vi "EV05故障解析.vi"() -> ()   [LabVIEW 2013]
panel:
  in  "选择故障类型":u32(ring) items=["电池故障", "硬件故障", "电池系统故障1", "电池系统故障2"]
  in  "输入故障码":string caption="输入故障码  (16位的十六进制数值)"
  in  "故码障解析123":bool
  out "电池故障":string[][](array[string])
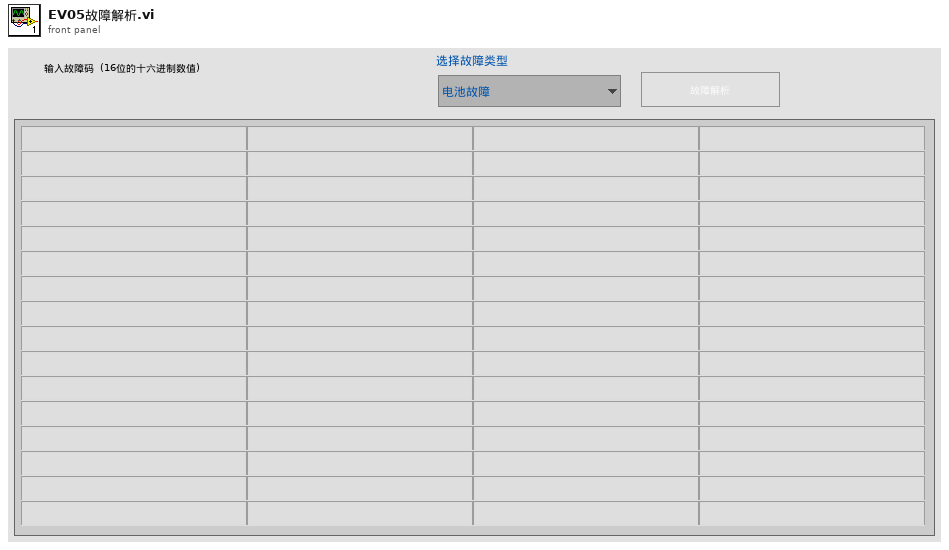
[diagram p1: front panel]
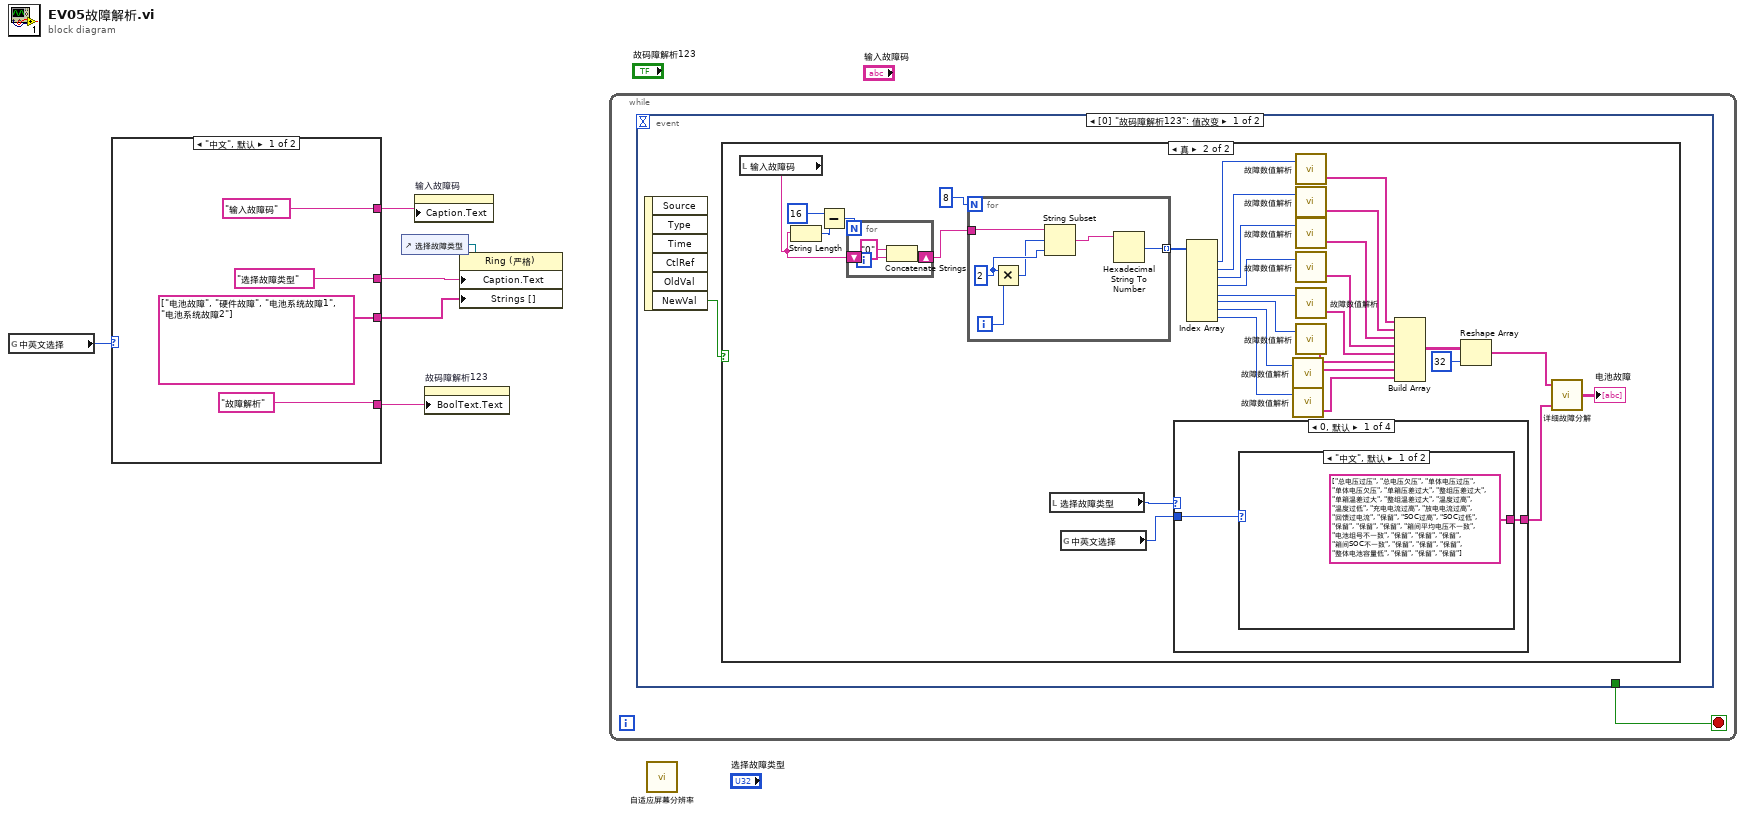
[diagram p0: block diagram]
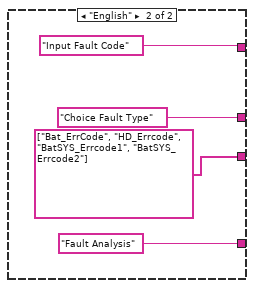
[diagram p2: hidden frame]
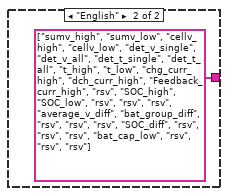
[diagram p4: hidden frame]
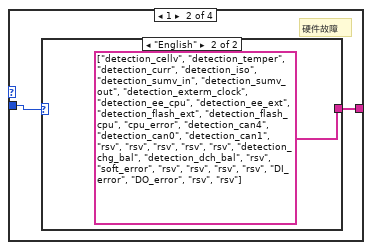
[diagram p5: hidden frame]
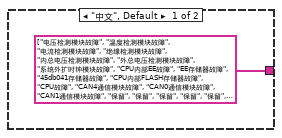
[diagram p6: hidden frame]
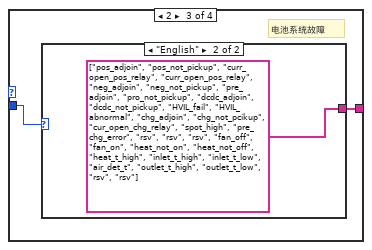
[diagram p7: hidden frame]
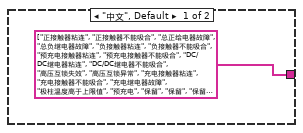
[diagram p8: hidden frame]
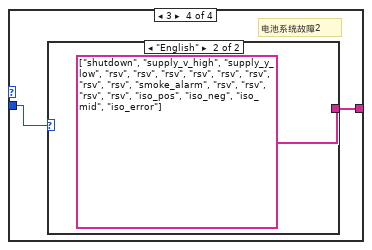
[diagram p9: hidden frame]
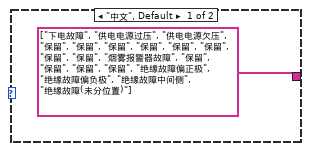
[diagram p10: hidden frame]
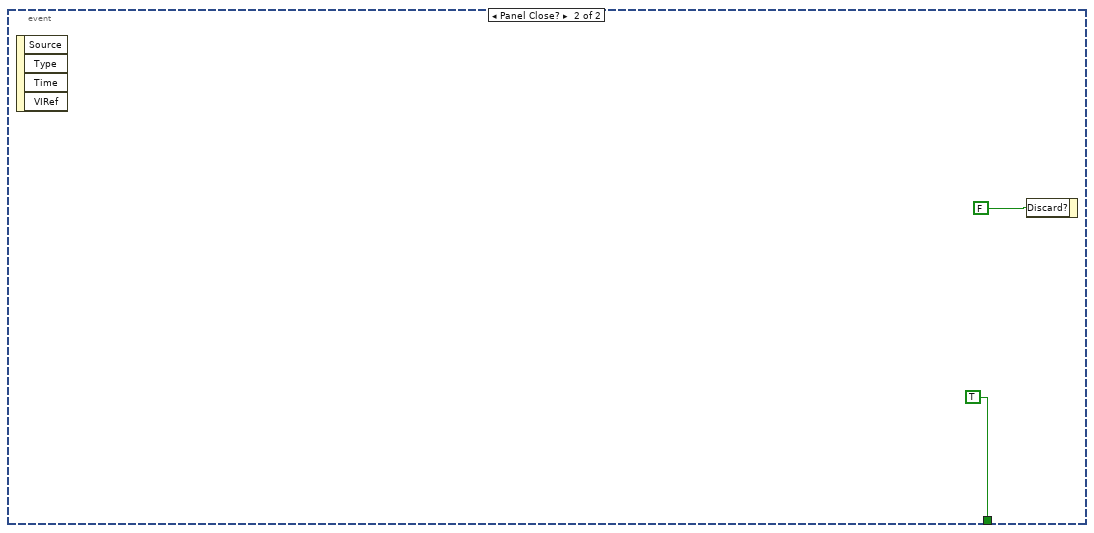
[diagram p11: hidden frame]
diagram:
  n1 = global read "中英文全局.vi" "中英文选择"() -> (w1:enum32{"中文", "English"})
  n2 = case shown="\"中文\", 默认" w1 {
    tunnel: ["输入故障码" "Input Fault Code"] -> w6
    tunnel: ["选择故障类型" "Choice Fault Type"] -> w4
    tunnel: [string[] ["电池故障", "硬件故障", "电池系统故障1", "电池系统故障2"] ("字符串[]") string[] ["Bat_ErrCode", "HD_Errcode", "BatSYS_Errcode1", "BatSYS_Errcode2"] ("字符串[]")] -> w3
    tunnel: ["故障解析" "Fault Analysis"] -> w2
    frame "中文", Default {
    }
    frame "English" {
    }
  }
  n3 = control-ref of="选择故障类型"() -> (w5:refnum<vi>)
  n4 = property on="输入故障码" class="Str"("Caption.Text"=w6) -> ()  [unwired: 2 in, 2 out]
  n5 = property on="故码障解析123" class="Bool (严格)"("BoolText.Text"=w2) -> ()  [unwired: 2 in, 2 out]
  n6 = property class="Ring (严格)"(reference=w5, "Caption.Text"=w4, "Strings []"=w3) -> ()  [unwired: 1 in, 2 out]
  n7 = while {
    stop <- w15 stop-if-true
    n8 = event shown="[0] \"故码障解析123\": 值改变" {
      selector: _ -> [_ _]
      dyn-events: _ -> [_ _]
      timeout: _ -> [_ _]
      tunnel: [_ TRUE] -> w15
      event "故码障解析123": Value Change {
        n9 = event-data() -> ("NewVal"=w16:bool)  [unwired: 1 in, 5 out]
        n10 = case shown="真" w16 {
          frame False {
          }
          frame True {
            n11 = local read "输入故障码"() -> (w19:string)
            n12 = String Length(string=w19) -> (length=w21:i32)
            n13 = Subtract(x=16, y=w21) -> (x-y=w23:i32)
            n14 = for {
              N: w23 -> [_]
              shift-right: [w47] -> w20
              shift-left: w19 -> [w49]
              n15 = Concatenate Strings("0" ("字符串"), w49) -> (w47:string)
            }
            n16 = for {
              N: 8 -> [_]
              tunnel: w20 -> [w55]
              tunnel: [w54] -> w34 mode=indexing
              i -> [w50]
              w52 = 2 ("x")
              n17 = Multiply(x=w52, y=w50) -> (x*y=w51:i32)
              n18 = String Subset(string=w55, offset (0)=w51, length (rest)=w52) -> (substring=w53:string)
              n19 = Hexadecimal String To Number(string=w53) -> (number=w54:u32)  [unwired: 2 in, 1 out]
            }
            n20 = local read "选择故障类型"() -> (w18:u32)
            n21 = global read "中英文全局.vi" "中英文选择"() -> (w17:enum32{"中文", "English"})
            n22 = case shown="0, 默认" w18 {
              tunnel: [w57 w61 w65 w69] -> w46
              tunnel: w17 -> [w56 w60 w64 w68]
              frame 0, Default {
                n23 = case shown="\"中文\", 默认" w56 {
                  tunnel: [string[] ["总电压过压", "总电压欠压", "单体电压过压", "单体电压欠压", "单箱压差过大", "整组压差过大", "单箱温差过大", "整组温差过大", "温度过高", "温度过低", "充电电流过高", "放电电流过高", "回馈过电流", "保留", "SOC过高", "SOC过低", "保留", "保留", "保留", "箱间平均电压不一致", "电池组号不一致", "保留", "保留", "保留", "箱间SOC不一致", "保留", "保留", "保留", "整体电池容量低", "保留", "保留", "保留"] ("名称") string[] ["sumv_high", "sumv_low", "cellv_high", "cellv_low", "det_v_single", "det_v_all", "det_t_single", "det_t_all", "t_high", "t_low", "chg_curr_high", "dch_curr_high", "Feedback_curr_high", "rsv", "SOC_high", "SOC_low", "rsv", "rsv", "rsv", "average_v_diff", "bat_group_diff", "rsv", "rsv", "rsv", "SOC_diff", "rsv", "rsv", "rsv", "bat_cap_low", "rsv", "rsv", "rsv"] ("名称")] -> w57
                  frame "中文", Default {
                  }
                  frame "English" {
                  }
                }
              }
              frame 1 {
                # "硬件故障"
                n24 = case shown="\"English\"" w60 {
                  tunnel: [string[] ["电压检测模块故障", "温度检测模块故障", "电流检测模块故障", "绝缘检测模块故障", "内总电压检测模块故障", "外总电压检测模块故障", "系统外扩时钟模块故障", "CPU内部EE故障", "EE存储器故障", "45db041存储器故障", "CPU内部FLASH存储器故障", "CPU故障", "CAN4通信模块故障", "CAN0通信模块故障", "CAN1通信模块故障", "保留", "保留", "保留", "保留", "保留", "充电均衡模块故障", "放电均衡模块故障", "保留", "软件故障", "保留", "保留", "保留", "保留", "DI模块故障", "DO模块故障", "保留", "保留"] ("名称") string[] ["detection_cellv", "detection_temper", "detection_curr", "detection_iso", "detection_sumv_in", "detection_sumv_out", "detection_exterm_clock", "detection_ee_cpu", "detection_ee_ext", "detection_flash_ext", "detection_flash_cpu", "cpu_error", "detection_can4", "detection_can0", "detection_can1", "rsv", "rsv", "rsv", "rsv", "rsv", "detection_chg_bal", "detection_dch_bal", "rsv", "soft_error", "rsv", "rsv", "rsv", "rsv", "DI_error", "DO_error", "rsv", "rsv"] ("名称")] -> w61
                  frame "中文", Default {
                  }
                  frame "English" {
                  }
                }
              }
              frame 2 {
                # "电池系统故障"
                n25 = case shown="\"English\"" w64 {
                  tunnel: [string[] ["正接触器粘连", "正接触器不能吸合", "总正给电器故障", "总负继电器故障", "负接触器粘连", "负接触器不能吸合", "预充电接触器粘连", "预充电接触器不能吸合", "DC/DC继电器粘连", "DC/DC继电器不能吸合", "高压互锁失效", "高压互锁异常", "充电接触器粘连", "充电接触器不能吸合", "充电继电器故障", "极柱温度高于上限值", "预充电", "保留", "保留", "保留", "风机堵路", "风机开路", "加热不能开启", "加热不能关闭", "加热器温度高于上限值", "进风口温度过高", "进风口温度过低", "进风口,出风口温差故障", "出风口温度过高", "出风口温度过低", "保留", "保留"] ("名称") string[] ["pos_adjoin", "pos_not_pickup", "curr_open_pos_relay", "curr_open_pos_relay", "neg_adjoin", "neg_not_pickup", "pre_adjoin", "pro_not_pickup", "dcdc_adjoin", "dcdc_not_pickup", "HVIL_fail", "HVIL_abnormal", "chg_adjoin", "chg_not_pcikup", "cur_open_chg_relay", "spot_high", "pre_chg_error", "rsv", "rsv", "rsv", "fan_off", "fan_on", "heat_not_on", "heat_not_off", "heat_t_high", "inlet_t_high", "inlet_t_low", "air_det_t", "outlet_t_high", "outlet_t_low", "rsv", "rsv"] ("名称")] -> w65
                  frame "中文", Default {
                  }
                  frame "English" {
                  }
                }
              }
              frame 3 {
                # "电池系统故障2"
                n26 = case shown="\"English\"" w68 {
                  tunnel: [string[] ["下电故障", "供电电源过压", "供电电源欠压", "保留", "保留", "保留", "保留", "保留", "保留", "保留", "保留", "烟雾报警器故障", "保留", "保留", "保留", "保留", "绝缘故障偏正极", "绝缘故障偏负极", "绝缘故障中间侧", "绝缘故障(未分位置)"] ("名称") string[] ["shutdown", "supply_v_high", "supply_y_low", "rsv", "rsv", "rsv", "rsv", "rsv", "rsv", "rsv", "rsv", "smoke_alarm", "rsv", "rsv", "rsv", "rsv", "iso_pos", "iso_neg", "iso_mid", "iso_error"] ("名称")] -> w69
                  frame "中文", Default {
                  }
                  frame "English" {
                  }
                }
              }
            }
            n27 = Index Array(array=w34) -> (element #1=w33:u32, element #2=w32:u32, element #3=w31:u32, element #4=w30:u32, element #5=w29:u32, element #6=w28:u32, element #7=w27:u32, element #8=w26:u32)  [unwired: 8 in]
            n28 = call "故障数值解析.vi"("输入"=w27) -> ("结果"=w40:string[])  [unwired: 2 out]
            n29 = call "故障数值解析.vi"("输入"=w26) -> ("结果"=w38:string[])  [unwired: 2 out]
            n30 = call "故障数值解析.vi"("输入"=w33) -> ("结果"=w45:string[])  [unwired: 2 out]
            n31 = call "故障数值解析.vi"("输入"=w32) -> ("结果"=w44:string[])  [unwired: 2 out]
            n32 = call "故障数值解析.vi"("输入"=w31) -> ("结果"=w43:string[])  [unwired: 2 out]
            n33 = call "故障数值解析.vi"("输入"=w30) -> ("结果"=w39:string[])  [unwired: 2 out]
            n34 = call "故障数值解析.vi"("输入"=w29) -> ("结果"=w42:string[])  [unwired: 2 out]
            n35 = call "故障数值解析.vi"("输入"=w28) -> ("结果"=w41:string[])  [unwired: 2 out]
            n36 = Build Array(w45, w44, w43, w39, w42, w41, w40, w38) -> (w36:string[][])
            n37 = Reshape Array(w36, 32 ("维数大小")) -> (w35:string[])
            n38 = call "详细故障分解.vi"("名称"=w46, "故障输入口"=w35) -> ("输出数组"=→"电池故障":string[][])  [unwired: 3 out]
          }
        }
      }
      event Panel Close? {
        n39 = event-data() -> ()  [unwired: 1 in, 4 out]
        n40 = event-data("Discard?"=FALSE) -> ()  [unwired: 1 in, 1 out]
      }
    }
  }
  n41 = call "自适应屏幕分辨率.vi"() -> ()  [unwired: 16 in]
